vi "Test Unicode Tag FLAC.vi"(8 "error in (no error)":errorcluster) -> (0 "error out":errorcluster, 3 "Pass?":bool)   [LabVIEW 2020]
uses:
  G-Audio/Controls/Text Encoding.ctl
  G-Audio/Audio Files/Polymorphic VIs/Get Audio File Tags (Path).vi
  G-Audio/G-Audio.lvlib
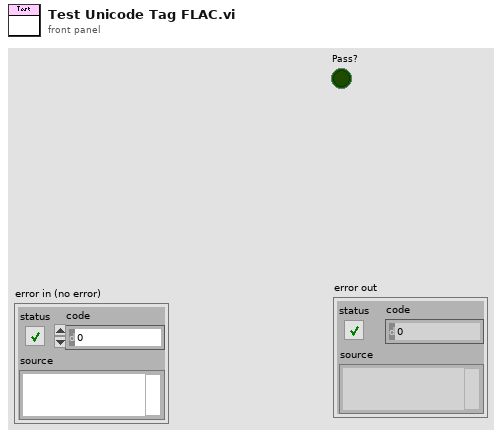
[diagram p1: front panel]
types:
  T1 = typedef "G-Audio.lvlib/Text Encoding.ctl" = enum16{"ASCII", "UTF-8", "UTF-16 LE"}
  T2 = typedef "G-Audio.lvlib/Audio File Tag.ctl" = cluster{"Field":string, "Value":string}
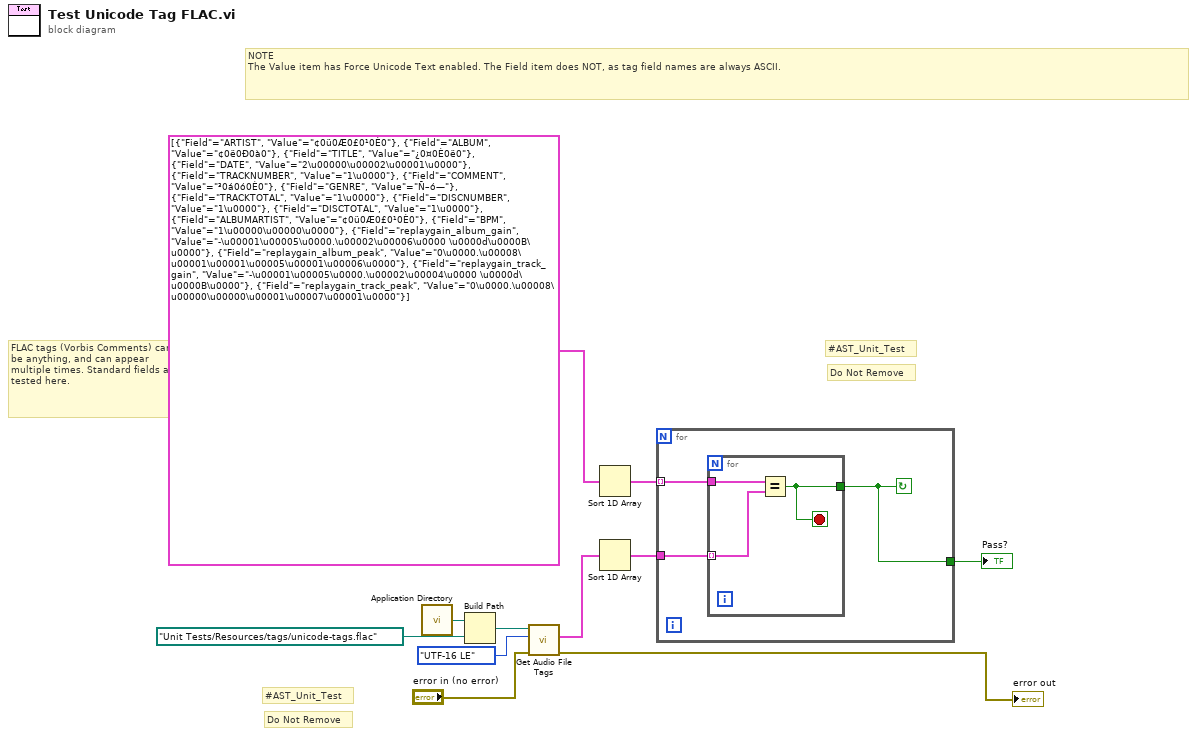
[diagram p0: block diagram]
diagram:
  # "NOTE\nThe Value item has Force Unicode Text enabled. The Field item does NOT, as tag field names are always ASCII."
  # "FLAC tags (Vorbis Comments) can be anything, and can appear multiple times. Standard fields are tested here."
  # "Do Not Remove"
  # "#AST_Unit_Test"
  # "Do Not Remove"
  # "#AST_Unit_Test"
  n1 = call <vilib>:"Application Directory.vi"() -> ("Application Directory"=w11:path)
  n2 = Build Path(base path=w11, name or relative path=path "Unit Tests/Resources/tags/unicode-tags.flac" ("Path")) -> (appended path=w9:path)
  n3 = call-poly "Get Audio File Tags.vi"("error in (no error)"="error in (no error)", "Encoding (ASCII)"=Text_Encoding."UTF-16 LE", "Path In"=w9) -> ("error out"=→"error out":errorcluster, "Tags"=w8:T2[])  [unwired: 5 in, 2 out]
  n4 = Sort 1D Array(array=cluster{"Field":string, "Value":string}[] [{"Field"="ARTIST", "Value"="¢0ü0Æ0£0¹0È0"}, {"Field"="ALBUM", "Value"="¢0ë0Ð0à0"}, {"Field"="TITLE", "Value"="¿0¤0È0ë0"}, {"Field"="DATE", "Value"="2\u00000\u00002\u00001\u0000"}, {"Field"="TRACKNUMBER", "Value"="1\u0000"}, {"Field"="COMMENT", "Value"="³0á0ó0È0"}, {"Field"="GENRE", "Value"="Ñ–ó—"}, {"Field"="TRACKTOTAL", "Value"="1\u0000"}, {"Field"="DISCNUMBER", "Value"="1\u0000"}, {"Field"="DISCTOTAL", "Value"="1\u0000"}, {"Field"="ALBUMARTIST", "Value"="¢0ü0Æ0£0¹0È0"}, {"Field"="BPM", "Value"="1\u00000\u00000\u0000"}, {"Field"="replaygain_album_gain", "Value"="-\u00001\u00005\u0000.\u00002\u00006\u0000 \u0000d\u0000B\u0000"}, {"Field"="replaygain_album_peak", "Value"="0\u0000.\u00008\u00001\u00001\u00005\u00001\u00006\u0000"}, {"Field"="replaygain_track_gain", "Value"="-\u00001\u00005\u0000.\u00002\u00004\u0000 \u0000d\u0000B\u0000"}, {"Field"="replaygain_track_peak", "Value"="0\u0000.\u00008\u00000\u00000\u00001\u00007\u00001\u0000"}]) -> (sorted array=w6:cluster{"Field":string, "Value":string}[])
  n5 = Sort 1D Array(array=w8) -> (sorted array=w7:T2[])
  n6 = for {
    tunnel: w7 -> [w14]
    tunnel: w6 -> [w12] mode=indexing
    tunnel: [w13] -> w3
    stop <- w13 continue-if-true
    n7 = for {
      tunnel: w14 -> [w15] mode=indexing
      tunnel: [w16] -> w13
      tunnel: w12 -> [w17]
      stop <- w16 stop-if-true
      n8 = Equal?(x=w17, y=w15) -> (x = y?=w16:bool)
    }
  }
  "Pass?" <- w3
